vi "SVFA Zoom Frequency Response (Mag-Phase).vi"(0 "stimulus signal X [EUx]":waveform(dbl)={"t0"=timestamp(0 s since 1904-01-01), "dt"=1e-05, "Y"=[]}, 1 "response signal Y [EUy]":waveform(dbl)={"t0"=timestamp(0 s since 1904-01-01), "dt"=1e-05, "Y"=[]}, 3 "zoom settings":T7={"frequency range"={"start frequency"=1000.0, "stop frequency"=2000.0}, "window"=1, "number of lines"=400, "% overlap"=0.0} {"% overlap" min=0.0 format="%.2f"; "number of lines" min=2; "window" items=["None ", "Hanning", "Hamming", "Blackman-Harris", "Exact Blackman", "Blackman", "Flat Top", "4 Term B-Harris ", "7 Term B-Harris", "Low Sidelobe"]; "frequency range"."stop frequency" min=0.0 format="%.2f"; "frequency range"."start frequency" min=0.0 format="%.2f"}, 4 "view":T9={"dB On (T)"=TRUE, "unwrap phase (F)"=FALSE, "convert to degree (T)"=TRUE}, 5 "error in (no error)":errorcluster, 6 "FRF mode":enum16{"H1", "H2", "H3"}(ring), 7 "averaging parameters":T8={"averaging mode"=enum."No averaging", "weighting mode"=enum."Exponential", "number of averages"=10, "linear mode"=enum."One shot"} {"number of averages" min=1 step=1}, 9 "restart averaging (F)":bool) -> (10 "new spectrum available":bool, 11 "averaging done":bool, 12 "coherence":cluster{"f0":dbl, "df":dbl, "coherence":dbl[]} {"coherence" format="%.2f"; "df" format="%.2f"; "f0" format="%.2f"}, 13 "averages completed":dbl, 14 "magnitude [dB EUy/EUx]":cluster{"f0":dbl, "df":dbl, "magnitude":dbl[]} {"magnitude" format="%.2f"; "df" format="%.2f"; "f0" format="%.2f"}, 15 "magnitude unit label":string, 16 "phase [degrees]":cluster{"f0":dbl, "df":dbl, "phase":dbl[]} {"phase" format="%.2f"; "df" format="%.2f"; "f0" format="%.2f"}, 17 "phase unit label":string, 18 "spectrum info":T1={"channel name"="", "description"="", "x-axis units"=1, "spectral info"={"spectrum type"=enum."Power [Magnitude^2]", "linear/dB"=enum."linear", "window"=0, "window size"=0, "FFT size"=0}, "engineering units"=0, "custom label"="", "dB reference [EU]"=0.0, "peak units"=enum."rms", "weighting filter"=0, "spectral density?"=FALSE, "unit label"="", "spectrum skewed?"=FALSE, "complimentary spectrum units"=enum."none"} {"x-axis units" items=["Time (s)"=0, "Frequency-CB (Hz)"=1, "Frequency-CPB (Hz)"=1248, "Frequency-Arbitrary (Hz)"=2357, "Quefrency (s)"=2, "Revolutions (rev)"=3, "Order"=4, "Speed (RPM)"=11, "Speed (rad/s)"=21, "Index"=65535]; "weighting filter" items=["Linear", "A-weighting", "B-weighting", "C-weighting", "ITU-R 468-4", "Dolby", "CCITT", "C-message", "Wb", "Wc", "Wd", "We", "Wf", "Wh", "Wj", "Wk", "Wm", "AES17 20 kHz lowpass", "AES17 40 kHz lowpass", "AES17 20 kHz highpass", "AES17 40 kHz highpass"]; "dB reference [EU]" format="%.2f"; "engineering units" items=["custom..."=0, "V"=1, "A"=21, "C"=30, "pC"=31, "s"=32, "-"=29, "Pa"=2, "N"=20, "g"=3, "m/s^2"=4, "m/s"=5, "m"=6, "mm/s"=12, "mm"=13, "micron/s"=14, "micron"=15, "in/s^2"=7, "in/s"=8, "in"=9, "mil/s"=10, "mil"=11, "rad/s^2"=16, "rad/s"=17, "rad"=18, "deg/s^2"=26, "deg/s"=27, "deg"=28, "RPM"=22, "cycle/s^2"=23, "Hz"=24, "cycle"=25, "strain"=19]; "spectral info"."window" items=["None "=0, "Hanning"=1, "Hamming"=2, "Blackman-Harris"=3, "Exact Blackman"=4, "Blackman"=5, "Flat Top"=6, "4 Term B-Harris "=7, "7 Term B-Harris"=8, "Low Sidelobe"=9, "Force - Exponential"=10, "Gaussian"=62]}, 19 "error out":errorcluster)   [LabVIEW 2017]
doc: "Computes the zoom frequency response and the coherence of <B>stimulus signal X [EUx]</B>, <B>response signal Y [EUy]</B>, and <B>zoom settings</B>. Results are returned in coherence, magnitude, and phase. Data accumulates each time this VI is called. However, it returns a new spectrum only when sufficient data accumulates. Indicators and subsequent processing should only be called when <B>new spectrum available</B> is TRUE.\n\nZoom frequency response is typically an averaged measurement."
uses:
  <vilib>/addons/_NISVFA/_Shared subVIs/Controls/svc_Spectrum Info.ctl
  <vilib>/addons/_NISVFA/_Shared subVIs/Controls/svc_X-Axis Units.ctl
  <vilib>/addons/_NISVFA/_Shared subVIs/Controls/svc_Spectrum Type.ctl
  <vilib>/addons/_NISVFA/_Shared subVIs/Controls/svc_Engineering Units Text Ring.ctl
  <vilib>/addons/_NISVFA/_Shared subVIs/Controls/svc_Weighting Filter Text Ring.ctl
  <vilib>/addons/_NISVFA/_Shared subVIs/Controls/svc_Complimentary Spectrum Units.ctl
  <vilib>/addons/_NISVFA/_Shared subVIs/Spectrum Averaging/svfa_Reset Averaging State Info.vi
  <vilib>/addons/_NISVFA/_Shared subVIs/Spectrum Averaging/svfa_Average Array with Avg Checks (complex) No State.vi
  <vilib>/addons/_NISVFA/_Shared subVIs/Spectrum Averaging/svfa_Average Spectrum (complex) No State.vi
  <vilib>/addons/_NISVFA/_Shared subVIs/Spectrum Averaging/svfa_Average Array (complex) No State.vi
  <vilib>/addons/_NISVFA/_Shared subVIs/Spectrum Averaging/svfa_No Average Array (complex).vi
  <vilib>/addons/_NISVFA/_Shared subVIs/Spectrum Averaging/svfa_Average Array (complex).vi
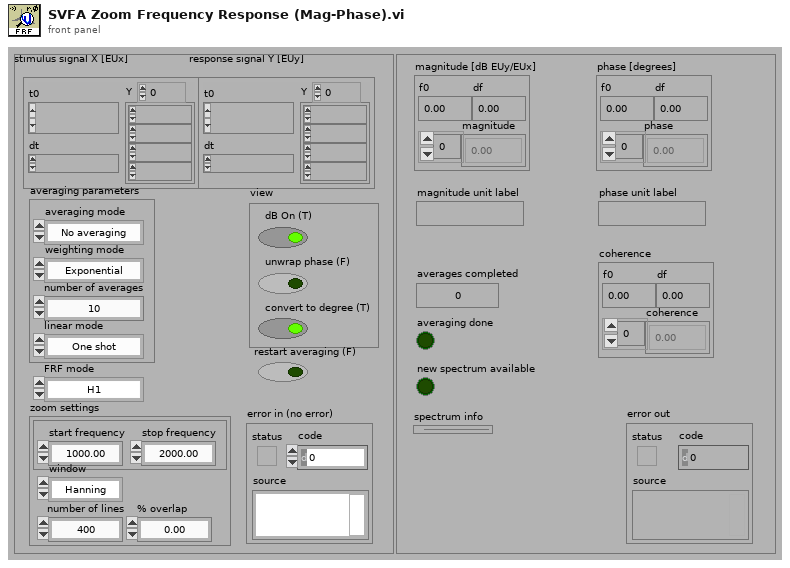
[diagram p1: front panel]
types:
  T1 = typedef "svc_Spectrum Info.ctl" = cluster{"channel name":string, "description":string, "x-axis units":T2, "spectral info":cluster{"spectrum type":T3, "linear/dB":enum16{"linear", "dB"}, "window":u16, "window size":i32, "FFT size":i32}, "engineering units":T4, "custom label":string, "dB reference [EU]":dbl, "peak units":enum16{"rms", "peak", "peak-peak"}, "weighting filter":T5, "spectral density?":bool, "unit label":string, "spectrum skewed?":bool, "complimentary spectrum units":T6}
  T2 = typedef "svc_X-Axis Units.ctl" = u16
  T3 = typedef "svc_Spectrum Type.ctl" = enum16{"FFT Spectrum [complex]", "Amplitude [Magnitude]", "Power [Magnitude^2]", "Cross Spectrum [complex]", "Frequency Response [Complex]"}
  T4 = typedef "svc_Engineering Units Text Ring.ctl" = u16
  T5 = typedef "svc_Weighting Filter Text Ring.ctl" = u16
  T6 = typedef "svc_Complimentary Spectrum Units.ctl" = enum16{"none", "radians", "degrees", "cycles", "imaginary"}
  T7 = cluster{"frequency range":cluster{"start frequency":dbl, "stop frequency":dbl}, "window":u16, "number of lines":i32, "% overlap":dbl}
  T8 = cluster{"averaging mode":enum16{"No averaging", "Vector averaging", "RMS averaging", "Peak hold"}, "weighting mode":enum16{"Linear", "Exponential"}, "number of averages":u32, "linear mode":enum16{"One shot", "Auto restart"}}
  T9 = cluster{"dB On (T)":bool, "unwrap phase (F)":bool, "convert to degree (T)":bool}
  T10 = enum16{"Restart processing", "Continue processing", "Skip processing"}
  T11 = enum16{"Cross spectrum", "Frequency response", "Coherent output power"}
  T12 = enum16{"No averaging", "Vector averaging", "RMS averaging", "Peak hold"}
  T13 = cluster{"zoom settings":cluster{"center frequency":dbl, "zoom":i32, "trim":dbl}, "FFT settings":cluster{"window":enum16{"None ", "Hanning", "Hamming", "Blackman-Harris", "Exact Blackman", "Blackman", "Flat Top", "4 Term B-Harris ", "7 Term B-Harris", "Low Sidelobe"}, "window size":i32, "FFT size":i32, "%overlap":dbl}}
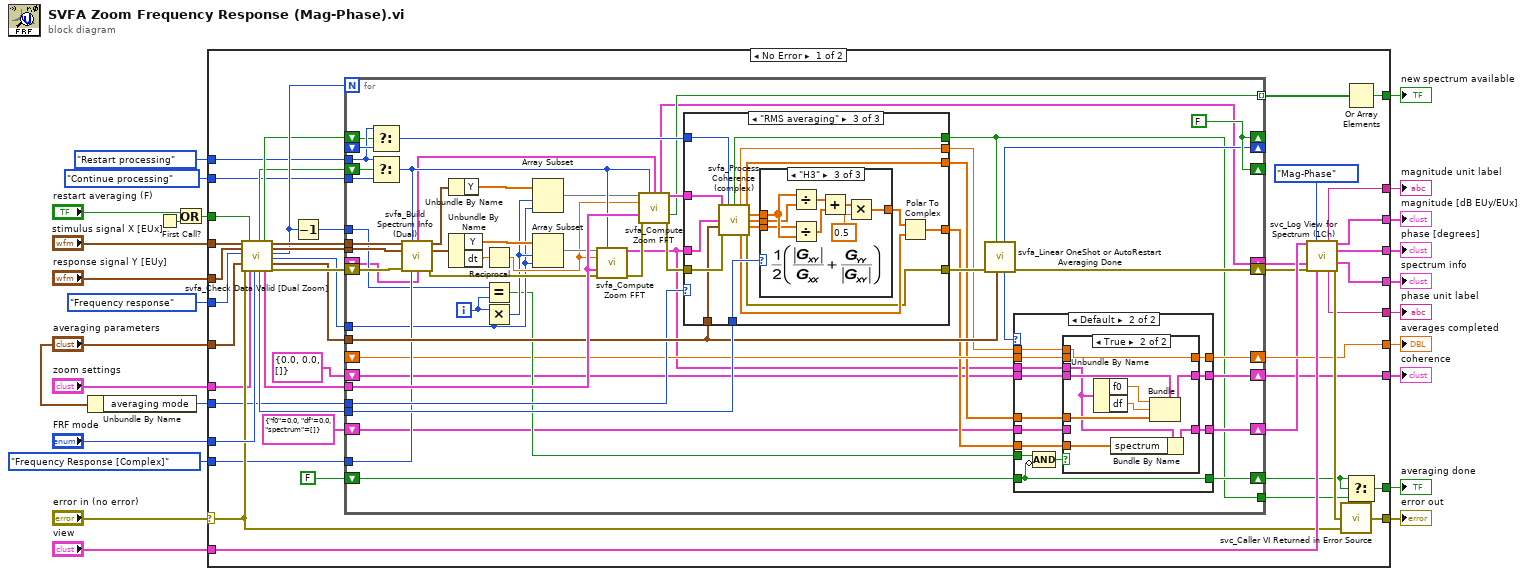
[diagram p0: block diagram]
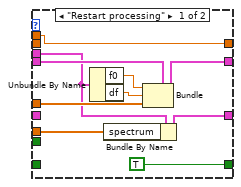
[diagram p2: hidden frame]
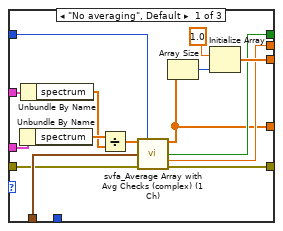
[diagram p4: hidden frame]
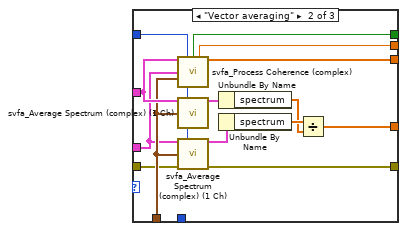
[diagram p5: hidden frame]
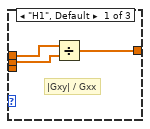
[diagram p6: hidden frame]
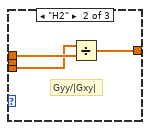
[diagram p7: hidden frame]
diagram:
  n1 = Unbundle By Name("averaging parameters") -> ("averaging mode"=w3:T12)
  n2 = First Call?() -> (First Call?: T/F=w9:bool)
  n3 = Or(x="restart averaging (F)", y=w9) -> (x .or. y?=w8:bool)
  n4 = case shown="No Error" "error in (no error)" {
    selector: "error in (no error)" -> [w57 w218]
    tunnel: "stimulus signal X [EUx]" -> [w70 _]
    tunnel: "response signal Y [EUy]" -> [w69 _]
    tunnel: [w66 _] -> w22
    tunnel: [w65 _] -> w21
    tunnel: [w49 _] -> w20
    tunnel: [w58 w218] -> w19
    tunnel: [w27 _] -> w18
    tunnel: w8 -> [w67 _]
    tunnel: "view" -> [w63 _]
    tunnel: "zoom settings" -> [w55 _]
    tunnel: [w29 _] -> w15
    tunnel: [w52 _] -> w14
    tunnel: [w64 _] -> w13
    tunnel: "FRF mode" -> [w62 _]
    tunnel: [w61 _] -> w11
    tunnel: [w59 _] -> w10
    tunnel: "averaging parameters" -> [w68 _]
    tunnel: T11."Frequency response" ("measurement") -> [w54 _]
    tunnel: svc_Spectrum_Type."Frequency Response [Complex]" ("spectrum type") -> [w39 _]
    tunnel: w3 -> [w38 _]
    tunnel: T10."Restart processing" ("processing control") -> [w35 _]
    tunnel: T10."Continue processing" ("processing control") -> [w34 _]
    frame No Error {
      n5 = call <vilib>:"svfa_Check Data Valid [Dual Zoom].vi"("stimulus [X]"=w70, "response [Y]"=w69, "measurement"=w54, "averaging parameters"=w68, "error in (no error)"=w57, "restart averaging (F)"=w67, "zoom settings"=w55, "FRF mode"=w62) -> ("reset processing"=w36:bool, "dup FRF mode"=w43:enum16{"H1", "H2", "H3"}, "restart averaging"=w37:bool, "zoom FFT settings"=w40:T13, "dup stimulus [X]"=w47:waveform(dbl), "dup response [Y]"=w46:waveform(dbl), "iterations"=w42:i32, "maximum block size"=w33:i32, "dup averaging parameters"=w44:T8, "error out"=w45:errorcluster)  [unwired: 2 in]
      n6 = Decrement(x=w42) -> (x-1=w41:i32)
      n7 = for {
        N: w42 -> [_]
        shift-left: cluster{"f0":dbl, "df":dbl, "Coherence":dbl[]} {"f0"=0.0, "df"=0.0, "Coherence"=[]} -> [w77]
        shift-right: [w81] -> w49
        shift-left: cluster{"f0":dbl, "df":dbl, "spectrum":cdb[]} {"f0"=0.0, "df"=0.0, "spectrum"=[]} ("FFT spectrum") -> [w76]
        shift-right: [w78] -> w51
        tunnel: w44 -> [w116]
        tunnel: [w71] -> w26
        tunnel: [w75] -> w53 mode=indexing
        tunnel: w43 -> [w118]
        tunnel: w46 -> [w112]
        tunnel: w47 -> [w113]
        shift-right: [w73] -> w50
        shift-left: _ -> [w72]
        shift-right: [w89] -> _
        shift-left: _ -> [w104]
        tunnel: w41 -> [w97]
        tunnel: w40 -> [w122]
        tunnel: w39 -> [w107]
        tunnel: w38 -> [w114]
        shift-right: [w123] -> w48
        shift-left: w45 -> [w108]
        shift-right: [w85] -> w52
        shift-left: _ -> [w84]
        shift-right: [w99] -> _
        shift-left: w37 -> [w102]
        shift-right: [w99] -> _
        shift-left: w36 -> [w106]
        tunnel: w35 -> [w103]
        tunnel: w34 -> [w105]
        tunnel: w33 -> [w90]
        shift-right: [w87] -> w28
        shift-left: FALSE ("restart averaging") -> [w86]
        i -> [w98]
        w99 = FALSE ("reset processing")
        n8 = Select(t=w103, s=w102, f=w104) -> (s? t:f=w100:T10)
        n9 = Select(t=w103, s=w106, f=w105) -> (s? t:f=w101:T10)
        n10 = call <vilib>:"svfa_Build Spectrum Info (Dual).vi"("scaled signal  X [EU]"=w113, "processing control"=w101, "scaled signal  Y [EU]"=w112, "error in (no error)"=w108, "spectrum type"=w107, "spectrum info in"=w72) -> ("spectrum info out"=w74:T1, "dup scaled signal  X [EU]"=w111:waveform(dbl), "dup scaled signal  Y [EU]"=w110:waveform(dbl), "error out"=w109:errorcluster)  [unwired: 5 in, 1 out]
        n11 = Unbundle By Name ("Get Waveform Components")(w111) -> ("Y"=w96:dbl[])
        n12 = Unbundle By Name ("Get Waveform Components")(w110) -> ("Y"=w94:dbl[], "dt"=w121:dbl)
        n13 = Reciprocal(x=w121) -> (1/x=w92:dbl)
        n14 = Equal?(x=w97, y=w98) -> (x = y?=w88:bool)
        n15 = Multiply(x=w98, y=w90) -> (x*y=w91:i32)
        n16 = Array Subset(array=w96, index=w91, length=w90) -> (w95:dbl[])
        n17 = Array Subset(array=w94, index=w91, length=w90) -> (w93:dbl[])
        n18 = call <vilib>:"svfa_Compute Zoom FFT.vi"("x"=w93, "processing control"=w101, "fs"=w92, "zoom FFT settings"=w122, "error in (no error)"=w109) -> ("FFT spectrum"=w79:cluster{"f0":dbl, "df":dbl, "spectrum":cdb[]}, "error out"=w120:errorcluster)  [unwired: 6 in, 3 out]
        n19 = call <vilib>:"svfa_Compute Zoom FFT.vi"("x"=w95, "processing control"=w101, "spectrum info"=w74, "fs"=w92, "zoom FFT settings"=w122, "error in (no error)"=w120) -> ("spectrum info out"=w73:T1, "FFT spectrum"=w117:cluster{"f0":dbl, "df":dbl, "spectrum":cdb[]}, "spectrum ready"=w75:bool, "error out"=w119:errorcluster)  [unwired: 5 in, 1 out]
        n20 = case shown="\"RMS averaging\"" w114 {
          tunnel: [w161 w177 w190] -> w115
          tunnel: w116 -> [w165 w181 w201]
          tunnel: [w164 w184 w199] -> w71
          tunnel: w117 -> [w172 w186 w191]
          tunnel: w79 -> [w168 w179 w192]
          tunnel: w119 -> [w162 w178 w202]
          tunnel: w118 -> [_ _ w200]
          tunnel: [w163 w183 w198] -> w83
          tunnel: w100 -> [w160 w180 w197]
          tunnel: [w167 w175 w189] -> w82
          tunnel: [w159 w174 w188] -> w80
          frame "No averaging", Default {
            n21 = Unbundle By Name(w168) -> ("spectrum"=w173:cdb[])
            n22 = Unbundle By Name(w172) -> ("spectrum"=w170:cdb[])
            n23 = Divide(x=w173, y=w170) -> (x/y=w166:cdb[])
            n24 = call <vilib>:"svfa_Average Array with Avg Checks (complex) (1 Ch).vi"("spectrum"=w166, "processing control"=w160, "averaging parameters"=w165, "error in (no error)"=w162) -> ("average spectrum"=w159:cdb[], "averaging done"=w164:bool, "averages completed"=w163:dbl, "error out"=w161:errorcluster)  [unwired: 7 in, 1 out]
            n25 = Array Size(array=w159) -> (size(s)=w169:i32)
            n26 = Initialize Array(1.0 ("overwrite value"), w169) -> (w167:dbl[])
          }
          frame "Vector averaging" {
            n27 = call <vilib>:"svfa_Process Coherence (complex).vi"("X FFT spectrum [Vrms]"=w186, "processing control"=w180, "Y FFT spectrum [Vrms]"=w179, "averaging parameters"=w181) -> ("averaging done"=w184:bool, "averages completed"=w183:dbl, "Coherence"=w175:dbl[])  [unwired: 4 in, 5 out]
            n28 = call <vilib>:"svfa_Average Spectrum (complex) (1 Ch).vi"("spectrum"=w186, "processing control"=w180, "averaging parameters"=w181) -> ("spectrum"=w185:cluster{"f0":dbl, "df":dbl, "spectrum":cdb[]})  [unwired: 8 in, 4 out]
            n29 = call <vilib>:"svfa_Average Spectrum (complex) (1 Ch).vi"("spectrum"=w179, "processing control"=w180, "averaging parameters"=w181, "error in (no error)"=w178) -> ("spectrum"=w176:cluster{"f0":dbl, "df":dbl, "spectrum":cdb[]}, "error out"=w177:errorcluster)  [unwired: 7 in, 3 out]
            n30 = Unbundle By Name(w185) -> ("spectrum"=w182:cdb[])
            n31 = Unbundle By Name(w176) -> ("spectrum"=w187:cdb[])
            n32 = Divide(x=w187, y=w182) -> (x/y=w174:cdb[])
          }
          frame "RMS averaging" {
            n33 = call <vilib>:"svfa_Process Coherence (complex).vi"("X FFT spectrum [Vrms]"=w191, "processing control"=w197, "Y FFT spectrum [Vrms]"=w192, "averaging parameters"=w201, "error in (no error)"=w202) -> ("averaging done"=w199:bool, "averages completed"=w198:dbl, "Coherence"=w189:dbl[], "MAG <Gxy>"=w195:dbl[], "<Gxx>"=w194:dbl[], "<Gyy>"=w193:dbl[], "PHASE <Gxy>"=w196:dbl[], "error out"=w190:errorcluster)  [unwired: 3 in]
            n34 = case shown="\"H3\"" w200 {
              tunnel: w193 -> [_ w207 w210]
              tunnel: [w206 w209 w217] -> w203
              tunnel: w194 -> [w204 _ w211]
              tunnel: w195 -> [w205 w208 w212]
              frame "H1", Default {
                # "|Gxy| / Gxx"
                n35 = Divide(x=w205, y=w204) -> (x/y=w206:dbl[])
              }
              frame "H2" {
                # "Gyy/|Gxy|"
                n36 = Divide(x=w207, y=w208) -> (x/y=w209:dbl[])
              }
              frame "H3" {
                n37 = Divide(x=w212, y=w211) -> (x/y=w213:dbl[])
                n38 = Divide(x=w210, y=w212) -> (x/y=w214:dbl[])
                n39 = Add(x=w213, y=w214) -> (x+y=w215:dbl[])
                n40 = Multiply(x=w215, y=0.5) -> (x*y=w217:dbl[])
              }
            }
            n41 = Polar To Complex(1:w196, 2:w203) -> (0:w188:cdb[])
          }
        }
        n42 = call <vilib>:"svfa_Linear OneShot or AutoRestart Averaging Done.vi"("averaging parameters"=w116, "averaging done"=w71, "error in (no error)"=w115) -> ("error out"=w123:errorcluster, "processing control"=w89:T10)  [unwired: 7 in]
        n43 = case shown="Default" w89 {
          tunnel: [TRUE ("restart averaging") w144] -> w87
          tunnel: w86 -> [_ w144]
          tunnel: w88 -> [_ w146]
          tunnel: [w132 w143] -> w85
          tunnel: w84 -> [_ w142]
          tunnel: w83 -> [w132 w141]
          tunnel: w82 -> [w131 w140]
          tunnel: w79 -> [w124 w134]
          tunnel: [w127 w139] -> w81
          tunnel: w77 -> [w128 w136]
          tunnel: w80 -> [w126 w137]
          tunnel: [w125 w138] -> w78
          tunnel: w76 -> [_ w135]
          frame "Restart processing" {
            n44 = Unbundle By Name(w124) -> ("f0"=w129:dbl, "df"=w130:dbl)
            n45 = Bundle By Name(cluster=w124, "spectrum"=w126) -> (w125:cluster{"f0":dbl, "df":dbl, "spectrum":cdb[]})
            n46 = Bundle(cluster=w128, "f0"=w129, "df"=w130, "Coherence"=w131) -> (w127:cluster{"f0":dbl, "df":dbl, "Coherence":dbl[]})
          }
          frame Default {
            n47 = Compound Arithmetic op=AND(w146, invert w144) -> (w145:bool)
            n48 = case shown="True" w145 {
              tunnel: [w149 w158] -> w143
              tunnel: w142 -> [w149 _]
              tunnel: w141 -> [_ w158]
              tunnel: w134 -> [_ w150]
              tunnel: w140 -> [_ w155]
              tunnel: [w148 w151] -> w139
              tunnel: [w147 w154] -> w138
              tunnel: w137 -> [_ w153]
              tunnel: w136 -> [w148 w152]
              tunnel: w135 -> [w147 _]
              frame False {
              }
              frame True {
                n49 = Unbundle By Name(w150) -> ("f0"=w156:dbl, "df"=w157:dbl)
                n50 = Bundle By Name(cluster=w150, "spectrum"=w153) -> (w154:cluster{"f0":dbl, "df":dbl, "spectrum":cdb[]})
                n51 = Bundle(cluster=w152, "f0"=w156, "df"=w157, "Coherence"=w155) -> (w151:cluster{"f0":dbl, "df":dbl, "Coherence":dbl[]})
              }
            }
          }
        }
      }
      n52 = call <vilib>:"svc_Log View for Spectrum (1Ch).vi"("complex spectrum"=w51, "View"=enum16{"Mag-Phase", "Real-Imaginary"}."Mag-Phase", "spectrum info in"=w50, "error in (no error)"=w48, "view"=w63) -> ("unit label [mag or real]"=w61:string, "magnitude or real"=w66:cluster{"f0":dbl, "df":dbl, dbl[]}, "phase or imag"=w65:cluster{"f0":dbl, "df":dbl, dbl[]}, "spectrum info out"=w64:T1, "unit label [phase or imag]"=w59:string, "error out"=w60:errorcluster)  [unwired: 5 in]
      n53 = call <vilib>:"svc_Caller VI Returned in Error Source.vi"("warning input to caller"=w57, "error in (no error)"=w60) -> ("error out"=w58:errorcluster)  [unwired: 3 in]
      n54 = Or Array Elements(Boolean array=w53) -> (logical OR=w29:bool)
      n55 = Select(t=w28, s=w28, f=w26) -> (s? t:f=w27:bool)
    }
    frame Error {
    }
  }
  "error out" <- w19
  "magnitude [dB EUy/EUx]" <- w22
  "phase [degrees]" <- w21
  "averaging done" <- w18
  "averages completed" <- w14
  "coherence" <- w20
  "new spectrum available" <- w15
  "spectrum info" <- w13
  "magnitude unit label" <- w11
  "phase unit label" <- w10
